vi "Write Owned Test Methods.vi"(10 "Owned Test Methods":map{string, path}(c390), 11 "LUnit Test Case In":refnum<class "LUnit Test Case.lvclass">) -> (3 "LUnit Test Case Out":refnum<class "LUnit Test Case.lvclass">)   [LabVIEW 2020, in "LUnit Test Case.lvclass"]
uses:
  LUnit Test Case.lvclass
  LUnit Test Case.lvclass/LUnit Test Case.ctl
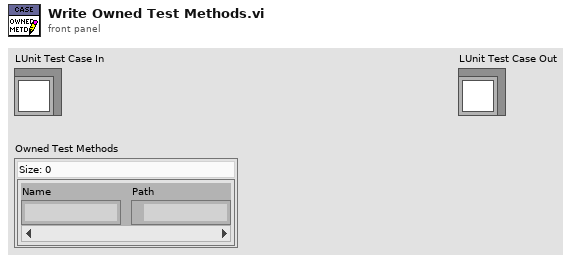
[diagram p1: front panel]
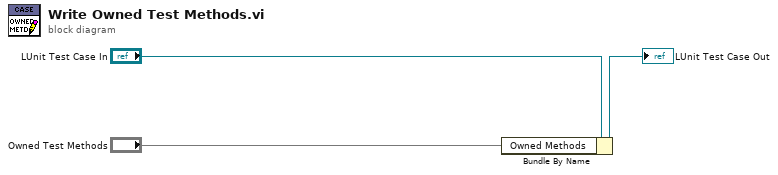
[diagram p0: block diagram]
diagram:
  n1 = Bundle By Name(cluster="LUnit Test Case In", "Owned Methods"="Owned Test Methods") -> (→"LUnit Test Case Out":refnum<class "LUnit Test Case.lvclass">)
